vi "Jens.vi"(9 "REPL":string, 10 "Send":string) -> ()   [LabVIEW 2020]
uses:
  <vilib>/Instr/_visa.llb/VISA Configure Serial Port (Instr).vi
panel:
  out "Cover":bool
  in  "Script":string
  in  "Buffer":string
  in  "Disconnect":bool
  in  "Help":bool
  in  "Connect":bool
  in  "Stop Button":bool
  in  "Port":refnum<visa-resource-name>
  out "Running Script":bool
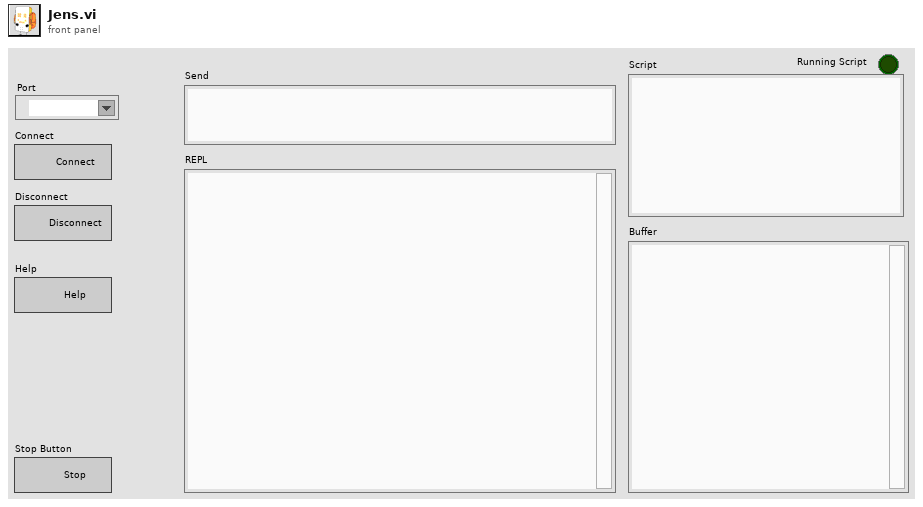
[diagram p1: front panel]
types:
  T1 = enum32{"Invalid", "Standard", "Closed", "Hidden", "Minimized", "Maximized"}
  T2 = typedef "eventvkey.ctl" = enum16{"ASCII", "Enter", "Return", "Shift", "Ctrl", "Alt", "Cmd", "Opt", "Caps", "NumLock", "Clear", "Break", "Up", "Down", "Left", "Right", "Insert", "Delete", "Home", "End", "PageUp", "PageDown", "Escape", "Help", "Pause", "ScrollLock", "F1", "F2", "F3", "F4", "F5", "F6", "F7", "F8", "F9", "F10", "F11", "F12", "F13", "F14", "F15", "F16", "F17", "F18", "F19", "F20", "F21", "F22", "F23", "F24", "Play", "VolumeUp", "VolumeDown", "Mute", "Two Byte Char"}
  T3 = cluster{"Shift":bool, "Ctrl":bool, "Alt":bool, "Cmd":bool, "Opt":bool}
  T4 = cluster{"Char":i16, "VKey":T2, "PlatMods":cluster{"Shift":bool, "Ctrl":bool, "Alt":bool, "Cmd":bool, "Opt":bool}}
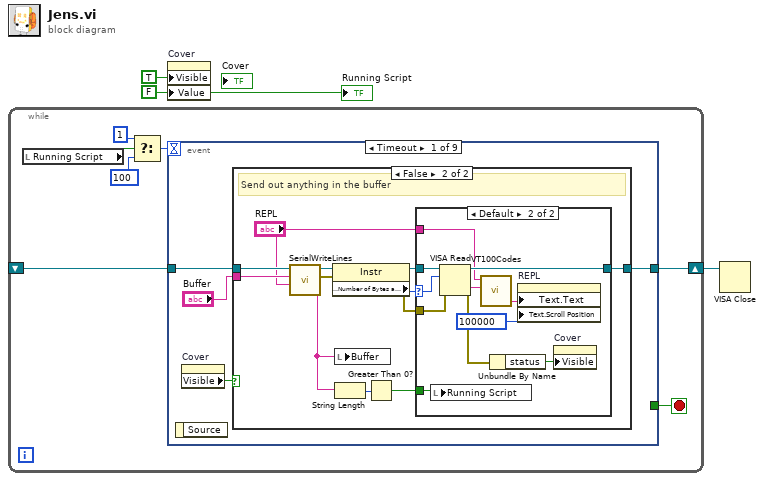
[diagram p0: block diagram]
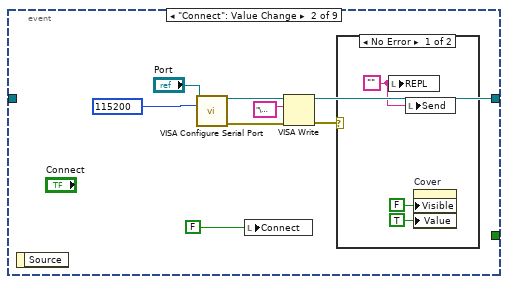
[diagram p4: hidden frame]
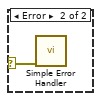
[diagram p5: hidden frame]
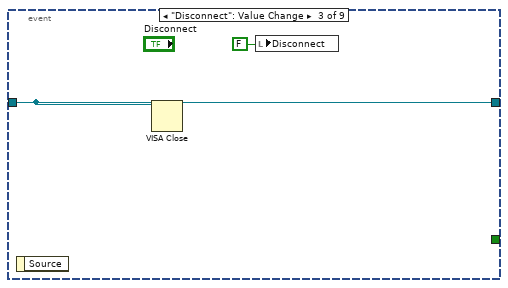
[diagram p6: hidden frame]
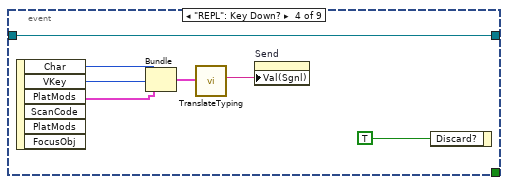
[diagram p7: hidden frame]
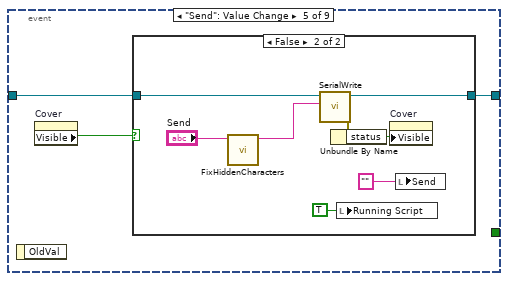
[diagram p8: hidden frame]
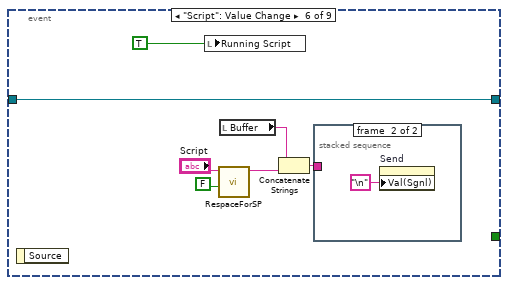
[diagram p10: hidden frame]
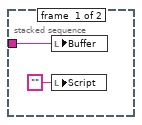
[diagram p11: hidden frame]
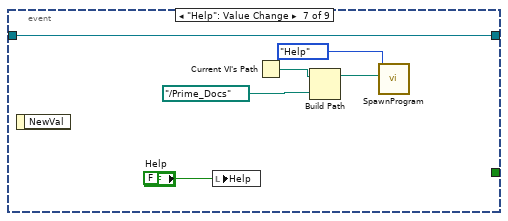
[diagram p12: hidden frame]
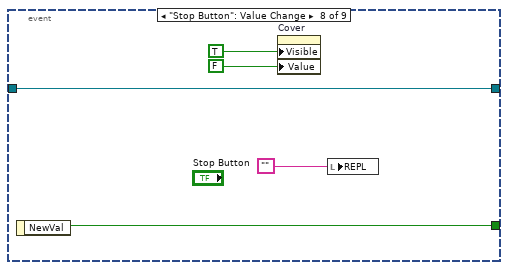
[diagram p13: hidden frame]
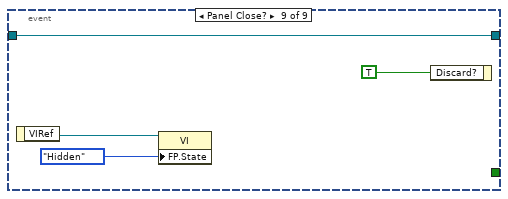
[diagram p14: hidden frame]
diagram:
  w1 = FALSE ("Cover")
  n1 = while {
    shift-right: [w9] -> w2
    shift-left: _ -> [w8]
    stop <- w10 stop-if-true
    n2 = local read "Running Script"() -> (w4:bool)
    n3 = Select(t=1, s=w4, f=100) -> (s? t:f=w5:i32)
    n4 = event shown="[0] Timeout" {
      selector: _ -> [_ _ _ _ _ _ _ _ _]
      dyn-events: _ -> [_ _ _ _ _ _ _ _ _]
      timeout: w5 -> [_ _ _ _ _ _ _ _ _]
      tunnel: [_ _ _ _ _ _ _ w90 _] -> w10
      tunnel: [w14 w43 w52 w59 w61 w76 w87 w91 w96] -> w9
      tunnel: w8 -> [w13 _ w52 w59 w62 w76 w87 w91 w96]
      event Timeout {
        n5 = event-data() -> ()  [unwired: 1 in, 1 out]
        n6 = property on="Cover" class="Bool (strict)"() -> ("Visible"=w12:bool)  [unwired: 2 in, 2 out]
        n7 = case shown="False" w12 {
          tunnel: [w15 w26] -> w14
          tunnel: w13 -> [w15 w25]
          tunnel: "Buffer" -> [_ w24]
          frame True {
          }
          frame False {
            # "Send out anything in the buffer"
            n8 = call "SerialWriteLines.vi"("REPL"="REPL", "Send"=w24, "VISA Refnum in"=w25) -> ("error out"=w21:errorcluster, "Rest"=w18:string, "VISA Refnum out"=w23:refnum<visa-resource-name>)  [unwired: 6 in]
            n9 = property class="Instr"(reference=w23, error in=w21) -> (error out=w20:errorcluster, "Serial Settings:Number of Bytes at Serial Port"=w22:u32)  [unwired: 1 out]
            n10 = local write "Buffer"(w18) -> ()
            n11 = String Length(string=w18) -> (length=w19:i32)
            n12 = Greater Than 0?(x=w19) -> (x > 0?=w17:bool)
            n13 = case shown="Default" w22 {
              selector: w22 -> [_ w34]
              tunnel: [w27 w38] -> w26
              tunnel: w23 -> [w27 w37]
              tunnel: w20 -> [_ w32]
              tunnel: w17 -> [_ w29]
              tunnel: "REPL" -> [_ w28]
              frame 0 {
              }
              frame Default {
                n14 = local write "Running Script"(w29) -> ()
                n15 = VISA Read(VISA resource name=w37, byte count=w34, error in (no error)=w32) -> (VISA resource name out=w38:refnum<visa-resource-name>, read buffer=w35:string, error out=w31:errorcluster)  [unwired: 1 out]
                n16 = call "VT100Codes.vi"("read buffer"=w35, "Console In"=w28) -> ("Console Out"=w33:string)  [unwired: 9 in]
                n17 = Unbundle By Name(w31) -> ("status"=w30:bool)
                n18 = property on="REPL" class="Str"("Text.Text"=w33, "Text.Scroll Position"=u32 100000 ("Text.Selection:Start")) -> ()  [unwired: 2 in, 2 out]
                n19 = property on="Cover" class="Bool (strict)"("Visible"=w30) -> ()  [unwired: 2 in, 2 out]
              }
            }
          }
        }
      }
      event "Connect": Value Change {
        n20 = event-data() -> ()  [unwired: 1 in, 1 out]
        n21 = call-poly "VISA Configure Serial Port"("VISA resource name"="Port", "baud rate (9600)"=u32 115200) -> ("VISA resource name out"=w44:refnum<visa-resource-name>, "error out"=w41:errorcluster)  [unwired: 12 in]
        n22 = local write "Connect"(FALSE ("Help")) -> ()
        n23 = VISA Write(VISA resource name=w44, write buffer="\u0003", error in (no error)=w41) -> (VISA resource name out=w43:refnum<visa-resource-name>, error out=w40:errorcluster)  [unwired: 1 out]
        n24 = case shown="No Error" w40 {
          selector: w40 -> [_ w50]
          frame No Error {
            w49 = ""
            n25 = local write "REPL"(w49) -> ()
            n26 = local write "Send"(w49) -> ()
            n27 = property on="Cover" class="Bool (strict)"("Visible"=FALSE, "Value"=TRUE ("Cover")) -> ()  [unwired: 2 in, 2 out]
          }
          frame Error {
            n28 = call <vilib>:"Simple Error Handler.vi"("error in (no error)"=w50) -> ()  [unwired: 4 in, 5 out]
          }
        }
      }
      event "Disconnect": Value Change {
        n29 = event-data() -> ()  [unwired: 1 in, 1 out]
        n30 = VISA Close(VISA resource name=w52) -> ()  [unwired: 1 in, 1 out]
        n31 = local write "Disconnect"(FALSE ("Help")) -> ()
      }
      event "REPL": Key Down? {
        n32 = event-data() -> ("Char"=w55:i16, "VKey"=w56:T2, "PlatMods"=w57:T3)  [unwired: 1 in, 3 out]
        n33 = Bundle("Char"=w55, "VKey"=w56, "PlatMods"=w57) -> (w58:T4)  [unwired: 1 in]
        n34 = call "TranslateTyping.vi"("Cluster"=w58) -> ("key"=w54:string)  [unwired: 10 in]
        n35 = property on="Send" class="Str"("Val(Sgnl)"=w54) -> ()  [unwired: 2 in, 2 out]
        n36 = event-data("Discard?"=TRUE) -> ()  [unwired: 1 in, 1 out]
      }
      event "Send": Value Change {
        n37 = event-data() -> ()  [unwired: 1 in, 1 out]
        n38 = property on="Cover" class="Bool (strict)"() -> ("Visible"=w60:bool)  [unwired: 2 in, 2 out]
        n39 = case shown="False" w60 {
          tunnel: w62 -> [w63 w71]
          tunnel: [w63 w70] -> w61
          frame True {
          }
          frame False {
            n40 = call "FixHiddenCharacters.vi"("String in"="Send") -> ("String out"=w64:string)  [unwired: 10 in]
            n41 = call "SerialWrite.vi"("Text"=w64, "VISA Refnum in"=w71) -> ("error out"=w66:errorcluster, "VISA Refnum out"=w70:refnum<visa-resource-name>)  [unwired: 8 in]
            n42 = Unbundle By Name(w66) -> ("status"=w65:bool)
            n43 = local write "Running Script"(TRUE ("Running Script")) -> ()
            n44 = property on="Cover" class="Bool (strict)"("Visible"=w65) -> ()  [unwired: 2 in, 2 out]
            n45 = local write "Send"("" ("Write text")) -> ()
          }
        }
      }
      event "Script": Value Change {
        n46 = event-data() -> ()  [unwired: 1 in, 1 out]
        n47 = local write "Running Script"(TRUE ("Visible")) -> ()
        n48 = call "RespaceForSP.vi"("Keep spaces?"=FALSE, "Code"="Script") -> ("Cleaned for SPIKE"=w73:string)  [unwired: 9 in]
        n49 = local read "Buffer"() -> (w74:string)
        n50 = Concatenate Strings(w74, w73) -> (w72:string)
        n51 = stacked-sequence {
          tunnel: w72 -> [w80 _]
          frame #0 {
            n52 = local write "Buffer"(w80) -> ()
            n53 = local write "Script"("" ("Script")) -> ()
          }
          frame #1 {
            n54 = property on="Send" class="Str"("Val(Sgnl)"="\n" ("Value (Signaling)")) -> ()  [unwired: 2 in, 2 out]
          }
        }
      }
      event "Help": Value Change {
        n55 = event-data() -> ()  [unwired: 1 in, 1 out]
        n56 = local write "Help"(FALSE ("Help")) -> ()
        n57 = Current VI's Path() -> (path=w85:path)
        n58 = Build Path(base path=w85, name or relative path=path "../Prime_Docs") -> (appended path=w83:path)
        n59 = call "SpawnProgram.vi"("Server"=w83, "Dialog"=enum16{"Help", "Files"}."Help") -> ()  [unwired: 10 in]
      }
      event "Stop Button": Value Change {
        n60 = event-data() -> ("NewVal"=w90:bool)  [unwired: 1 in]
        n61 = property on="Cover" class="Bool (strict)"("Visible"=TRUE, "Value"=FALSE ("Cover")) -> ()  [unwired: 2 in, 2 out]
        n62 = local write "REPL"("") -> ()
      }
      event Panel Close? {
        n63 = event-data() -> ("VIRef"=w94:refnum<vi>)  [unwired: 1 in]
        n64 = property class="VI"(reference=w94, "FP.State"=T1."Hidden" ("Front Panel Window:State")) -> ()  [unwired: 1 in, 2 out]
        n65 = event-data("Discard?"=TRUE) -> ()  [unwired: 1 in, 1 out]
      }
    }
  }
  n66 = property on="Cover" class="Bool (strict)"("Visible"=TRUE, "Value"=w1) -> ()  [unwired: 2 in, 2 out]
  n67 = VISA Close(VISA resource name=w2) -> ()  [unwired: 1 in, 1 out]
  "Running Script" <- w1
